vi "setUp.vi"(8 "error in (no error)":errorcluster, 11 "reference in":refnum<class "Test Unpause Timer.lvclass">) -> (0 "error out":errorcluster, 3 "reference out":refnum<class "Test Unpause Timer.lvclass">)   [LabVIEW 2018, in "Test Unpause Timer.lvclass"]
doc: "setUp runs prior to the test method during test execution. Use this method to initialize any object data required by your tests."
uses:
  Test Unpause Timer.lvclass
  C:/Program Files (x86)/National Instruments/LabVIEW 2018/vi.lib/addons/_JKI Toolkits/VI Tester/TestCase.llb/TestCase.lvclass
  Test Unpause Timer.lvclass/Test Unpause Timer.ctl
  <vilib>/addons/_JKI Toolkits/VI Tester/TestCase.llb/TestCase.lvclass
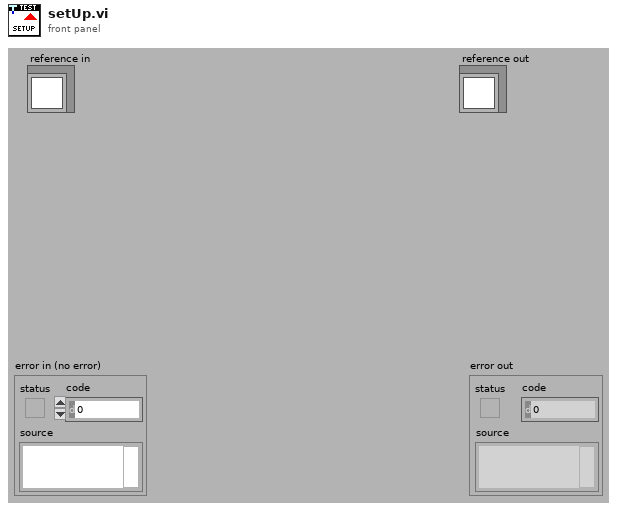
[diagram p1: front panel]
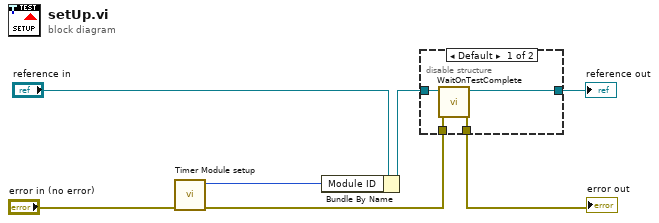
[diagram p0: block diagram]
diagram:
  n1 = call "Timer Module setup.vi"("error in (no error)"="error in (no error)") -> ("error out"=w1:errorcluster, "Module ID"=w3:i32)  [unwired: 9 in]
  n2 = Bundle By Name(cluster="reference in", "Module ID"=w3) -> (w4:refnum<class "Test Unpause Timer.lvclass">)
  n3 = disable-structure shown="Default" {
    disable-tunnel: w1 -> [w11 w12]
    disable-tunnel: [w10 w12] -> w7
    disable-tunnel: [w9 w13] -> w5
    disable-tunnel: w4 -> [w8 w13]
    frame condition #0 (active) {
      n4 = call <vilib>:"WaitOnTestComplete.vi"("error in (no error)"=w11, "TestCase in"=w8) -> ("error out"=w10:errorcluster, "TestCase out"=w9:refnum<class "Test Unpause Timer.lvclass">)  [unwired: 8 in]
    }
    frame condition #1 {
    }
  }
  "error out" <- w7
  "reference out" <- w5
